vi "ApplySmoothing.vi"(9 "Smoothing":u16(ring) items=["No smoothing"=0, "1/4 semitone"=25, "1/2 semitone"=50, "1 semitone"=100, "2 semitones"=200, "Woodhouse"=19], 11 "Complex FRF":cluster{dbl, "df":dbl, cdb[]}[](array[cluster])) -> (3 "Complex FRF Out":cluster{dbl, "df":dbl, cdb[]}[](array[cluster]))   [LabVIEW 2022 SP3]
uses:
  <vilib>/Analysis/4window.llb/Hanning Window (CDB).vi
  <vilib>/Analysis/4window.llb/AllCosWindow (CDB).vi
  <vilib>/Analysis/baseanly.llb/Mean (CDB).vi
  <vilib>/Analysis/NI_AALBase.lvlib
  <vilib>/Analysis/NI_AALPro.lvlib
panel:
  out "FRF Out 2":cluster{dbl, "df":dbl, dbl[]}[](graph)
  out "FRF In":cluster{dbl, "df":dbl, dbl[]}[](graph)
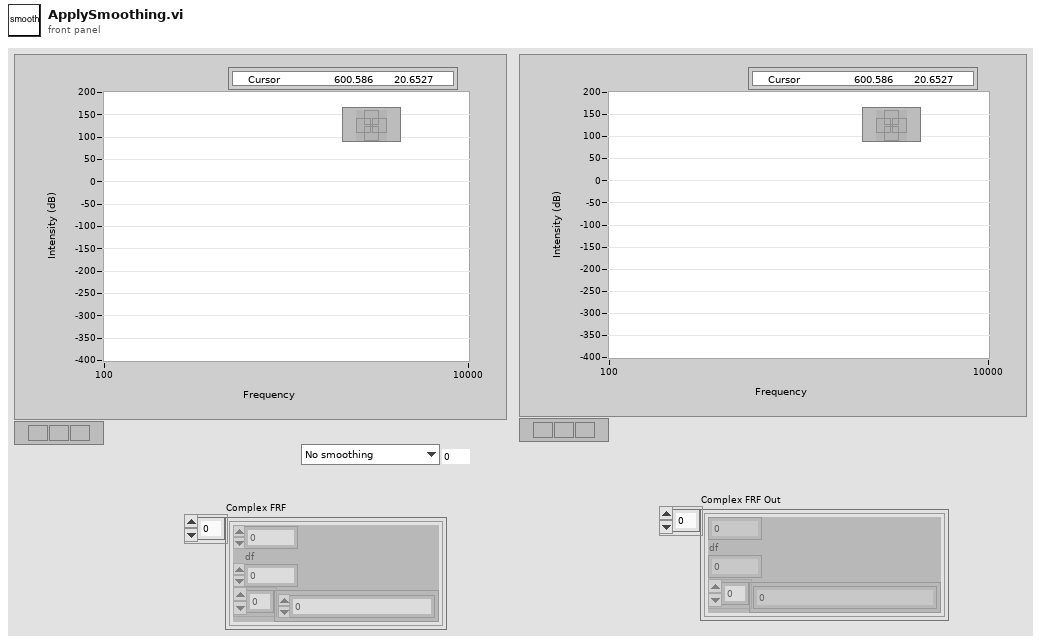
[diagram p1: front panel]
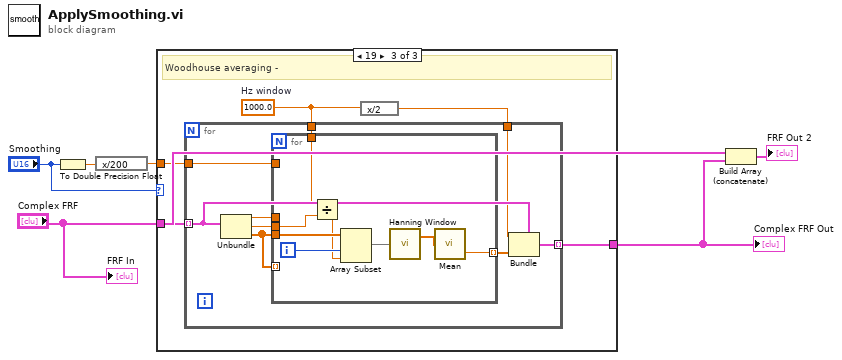
[diagram p0: block diagram]
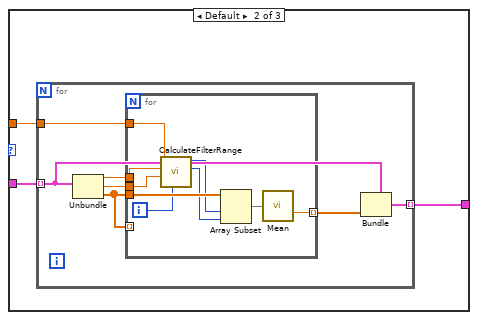
[diagram p3: hidden frame]
diagram:
  n1 = To Double Precision Float(number="Smoothing") -> (double precision float=w5:dbl)
  n2 = expression code="x/200"(w5) -> (w6:dbl)
  n3 = case shown="19" "Smoothing" {
    tunnel: w6 -> [_ w10 w31]
    tunnel: "Complex FRF" -> [w7 w9 w30]
    tunnel: [w7 w8 w29] -> w2
    frame 0 {
    }
    frame Default {
      n4 = for {
        tunnel: w9 -> [w13] mode=indexing
        tunnel: w10 -> [w15]
        tunnel: [w11] -> w8 mode=indexing
        n5 = Unbundle(w13) -> (w16:dbl, "df"=w17:dbl, w14:cdb[])
        n6 = for {
          tunnel: w17 -> [w19]
          tunnel: w16 -> [w20]
          tunnel: w14 -> [_] mode=indexing
          tunnel: w15 -> [w26]
          tunnel: w14 -> [w25]
          tunnel: [w22] -> w12 mode=indexing
          i -> [w21]
          n7 = call "CalculateFilterRange.vi"("n"=w21, "df"=w19, "f_0"=w20, "Semitone"=w26) -> ("range"=w24:i32, "start"=w18:i32)  [unwired: 6 in]
          n8 = Array Subset(array=w25, index=w18, length=w24) -> (w23:cdb[])
          n9 = call-poly <vilib>:"Mean.vi"("X"=w23) -> ("mean"=w22:cdb)  [unwired: 1 out]
        }
        n10 = Bundle(cluster=w13, w12) -> (w11:cluster{dbl, "df":dbl, cdb[]})  [unwired: 2 in]
      }
    }
    frame 19 {
      w28 = 1000.0  # Hz window
      # "Woodhouse averaging -"
      n11 = expression code="x/2"(w28) -> (w27:dbl)
      n12 = for {
        tunnel: w30 -> [w36] mode=indexing
        tunnel: w31 -> [w38]
        tunnel: [w34] -> w29 mode=indexing
        tunnel: w28 -> [w33]
        tunnel: w27 -> [w32]
        n13 = Unbundle(w36) -> (w39:dbl, "df"=w40:dbl, w37:cdb[])
        n14 = for {
          tunnel: w40 -> [w43]
          tunnel: w39 -> [_]
          tunnel: w37 -> [_] mode=indexing
          tunnel: w38 -> [_]
          tunnel: w37 -> [w48]
          tunnel: [w47] -> w35 mode=indexing
          tunnel: w33 -> [w41]
          i -> [w46]
          n15 = Divide(x=w41, y=w43) -> (x/y=w42:dbl)
          n16 = Array Subset(array=w48, index=w46, length=w42) -> (w45:cdb[])
          n17 = call-poly <vilib>:"Hanning Window.vi"("X"=w45) -> ("Windowed X"=w44:cdb[])  [unwired: 1 out]
          n18 = call-poly <vilib>:"Mean.vi"("X"=w44) -> ("mean"=w47:cdb)  [unwired: 1 out]
        }
        n19 = Bundle(cluster=w36, w32, w35) -> (w34:cluster{dbl, "df":dbl, cdb[]})  [unwired: 1 in]
      }
    }
  }
  "Complex FRF Out" <- w2
  n20 = Build Array (concatenate)("Complex FRF", w2) -> (→"FRF Out 2":cluster{dbl, "df":dbl, cdb[]}[])
  "FRF In" <- "Complex FRF"
